vi "2 bit Counter for FIFO U256.vi"(7 "Phase":fxp<+,2,2>=3.0, 8 "Increment?":bool, 11 "Reset?":bool) -> (0 "Phase Match?":bool, 3 "counter value":fxp<+,2,2>)   [LabVIEW 2012]
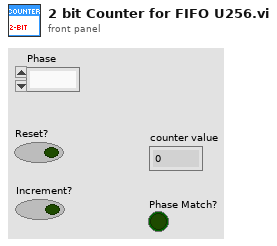
[diagram p1: front panel]
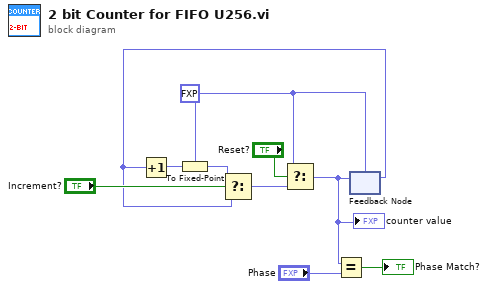
[diagram p0: block diagram]
diagram:
  w5 = fxp<+,2,2> 0.0 ("Counter FXP Type")
  n1 = feedback #1(w5) -> (w2:fxp<+,2,2>)
  n2 = Increment(x=w2) -> (x+1=w10:fxp<+,3,3>)
  n3 = To Fixed-Point(fixed-point type=w5, number=w10) -> (fixed-point=w9:fxp<+,2,2>)
  n4 = Select(t=w9, s="Increment?", f=w2) -> (s? t:f=w6:fxp<+,2,2>)
  n5 = Select(t=w5, s="Reset?", f=w6) -> (s? t:f=w1:fxp<+,2,2>)
  "counter value" <- w1
  n6 = Equal?(x=w1, y="Phase") -> (x = y?=→"Phase Match?":bool)
  n7 = feedback-in #1(w1) -> ()
